vi "Convert Array_Int to String.vi"(10 "Data 2":i32[][](array[numeric]), 11 "Data 1":i32[](array[numeric])) -> (3 "String Out":string)   [LabVIEW 2020, in "GUCalibration2.lvlib"]
uses:
  GUCalibration2.lvlib
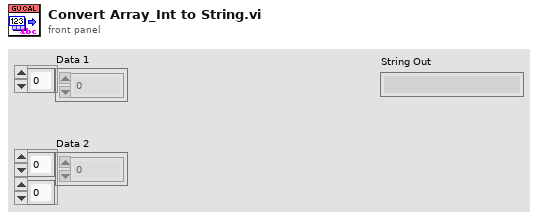
[diagram p1: front panel]
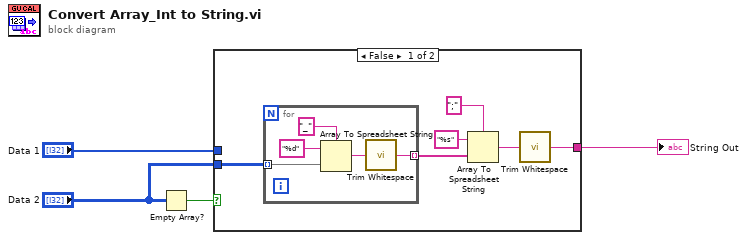
[diagram p0: block diagram]
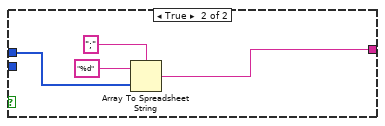
[diagram p2: hidden frame]
diagram:
  n1 = Empty Array?(array="Data 2") -> (empty?=w1:bool)
  n2 = case shown="False" w1 {
    tunnel: "Data 1" -> [_ w19]
    tunnel: "Data 2" -> [w10 _]
    tunnel: [w6 w17] -> w2
    frame False {
      n3 = for {
        tunnel: w10 -> [w14] mode=indexing
        tunnel: [w12] -> w7 mode=indexing
        n4 = Array To Spreadsheet String(delimiter (Tab)="_", array=w14, 3:"%d" ("format string")) -> (spreadsheet string=w13:string)
        n5 = call <vilib>:"Trim Whitespace.vi"("string"=w13) -> ("trimmed string"=w12:string)  [unwired: 1 in]
      }
      n6 = Array To Spreadsheet String(delimiter (Tab)=";", array=w7, 3:"%s" ("format string")) -> (spreadsheet string=w8:string)
      n7 = call <vilib>:"Trim Whitespace.vi"("string"=w8) -> ("trimmed string"=w6:string)  [unwired: 1 in]
    }
    frame True {
      n8 = Array To Spreadsheet String(delimiter (Tab)=";", array=w19, 3:"%d" ("format string")) -> (spreadsheet string=w17:string)
    }
  }
  "String Out" <- w2
